vi "MarkPlayersPosition.vi"(8 "error in (no error)":errorcluster, 9 "Player2NewPosition":T1, 10 "Player1NewPosition":T1, 11 "Board in":refnum<class "Board.lvclass">) -> (0 "error out":errorcluster, 1 "Player2AlreadyOccupied":bool, 2 "Player1AlreadyOccupied":bool, 3 "Board out":refnum<class "Board.lvclass">)   [LabVIEW 2015, in "TronviewGame.lvlib" / "Board.lvclass"]
uses:
  Board.lvclass
  Position.ctl
  BoardSize.ctl
  FieldState.ctl
  Board.lvclass/Board.ctl
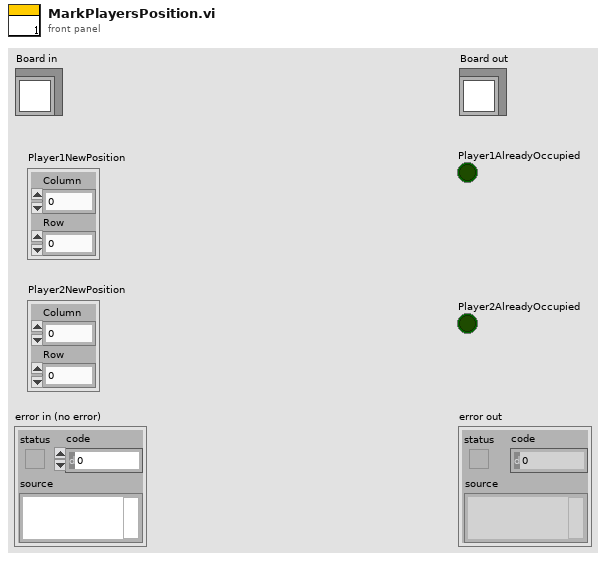
[diagram p1: front panel]
types:
  T1 = typedef "TronviewGame.lvlib/Board.lvclass/Position.ctl" = cluster{"Column":i32, "Row":i32}
  T2 = typedef "TronviewGame.lvlib/Board.lvclass/FieldState.ctl" = enum16{"Empty", "Blocked", "Player1Position", "Player2Postion", "Player1Marked", "Player2Marked"}
  T3 = typedef "TronviewGame.lvlib/Board.lvclass/BoardSize.ctl" = cluster{"Columns":u32, "Rows":u32}
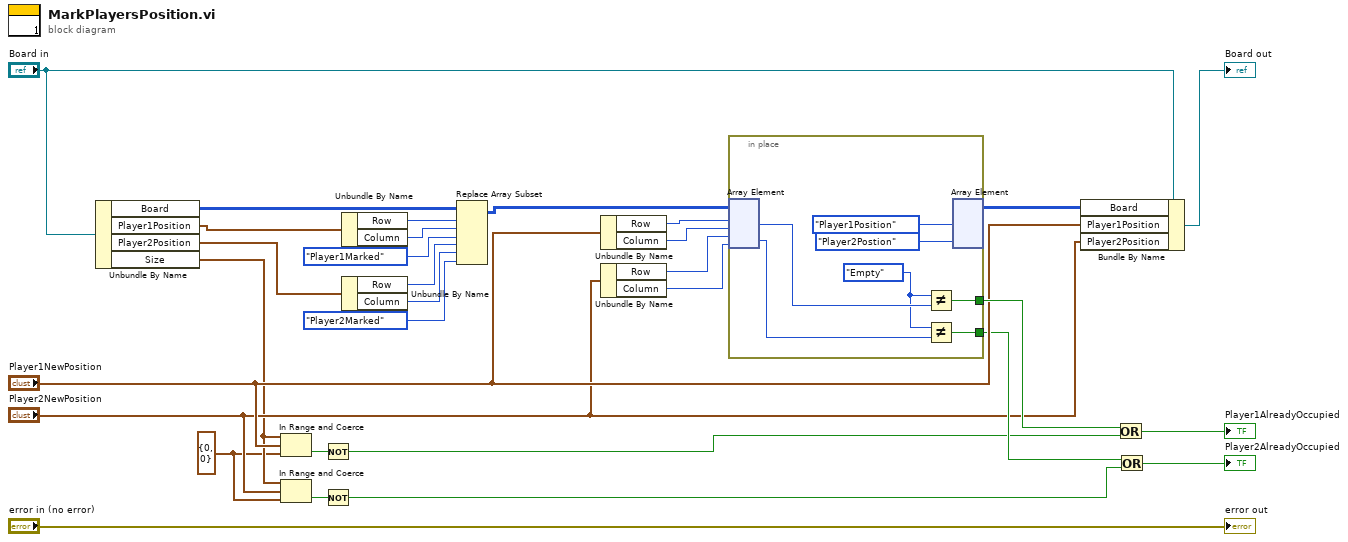
[diagram p0: block diagram]
diagram:
  w7 = T3 {"Columns"=0, "Rows"=0} ("lower limit")
  n1 = Unbundle By Name("Board in") -> ("Board"=w19:T2[][], "Player1Position"=w18:T1, "Player2Position"=w13:T1, "Size"=w8:T3)
  n2 = In Range and Coerce(upper limit=w8, x="Player1NewPosition", lower limit=w7) -> (In Range?=w3:bool)  [unwired: 1 out]
  n3 = In Range and Coerce(upper limit=w8, x="Player2NewPosition", lower limit=w7) -> (In Range?=w5:bool)  [unwired: 1 out]
  n4 = Not(x=w3) -> (.not. x?=w2:bool)
  n5 = Not(x=w5) -> (.not. x?=w1:bool)
  n6 = Unbundle By Name(w18) -> ("Row"=w24:i32, "Column"=w23:i32)
  n7 = Unbundle By Name(w13) -> ("Row"=w15:i32, "Column"=w14:i32)
  n8 = Replace Array Subset(array=w19, new element #1=FieldState."Player1Marked" ("element"), index (row) #1=w24, index (col) #1=w23, new element #2=FieldState."Player2Marked" ("element"), index (row) #2=w15, index (col) #2=w14) -> (w17:T2[][])
  n9 = Unbundle By Name("Player1NewPosition") -> ("Row"=w29:i32, "Column"=w28:i32)
  n10 = Unbundle By Name("Player2NewPosition") -> ("Row"=w12:i32, "Column"=w11:i32)
  n11 = in-place {
    in-place-border: [w34] -> w25
    in-place-border: [w31] -> w10
    w32 = FieldState."Empty" ("x")
    n12 = in-place-array #1(w17, w29, w28, w12, w11) -> (w37:T2, w33:T2)
    n13 = Not Equal?(x=w32, y=w37) -> (x != y?=w34:bool)
    n14 = Not Equal?(x=w32, y=w33) -> (x != y?=w31:bool)
    n15 = in-place-array #1(FieldState."Player1Position" ("element"), FieldState."Player2Postion" ("element")) -> (w26:T2[][])  [unwired: 4 out]
  }
  n16 = Bundle By Name(cluster="Board in", "Board"=w26, "Player1Position"="Player1NewPosition", "Player2Position"="Player2NewPosition") -> (→"Board out":refnum<class "Board.lvclass">)
  n17 = Or(x=w25, y=w2) -> (x .or. y?=→"Player1AlreadyOccupied":bool)
  n18 = Or(x=w10, y=w1) -> (x .or. y?=→"Player2AlreadyOccupied":bool)
  "error out" <- "error in (no error)"
